vi "replace plot - plot ref - V2.vi"(0 "Plot ref in":refnum<vi>, 1 "Array X IN":dbl[](array[numeric]), 2 "Array Y IN":dbl[](array[numeric]), 5 "plot index":i32, 6 "cursor action":T2=enum."write", 7 "label":enum16{"hide", "show x", "show y", "show (x,y)"}(ring), 12 "Color Box":u32(colorbox)=327424, 13 "cursor state":T3=enum."boring") -> (14 "Plot ref out":refnum<vi>, 15 "Array X":dbl[](array[numeric]), 16 "Array Y":dbl[](array[numeric]), 19 "2Dwindow bounds out":T1={"min y"=0.0021014740628288917, "max x"=44850.89441339177, "min x"=2.5658109925320947, "max y"=17480.201988350764} {"max y" format="%#9_9f"; "min x" format="%#9_9f"; "max x" format="%#9_9f"})   [LabVIEW 2020]
uses:
  cursor sate.ctl
  cursor action.ctl
  2Dwindow-bounds.ctl
  stack action -- control.ctl
  range multiplier action.ctl
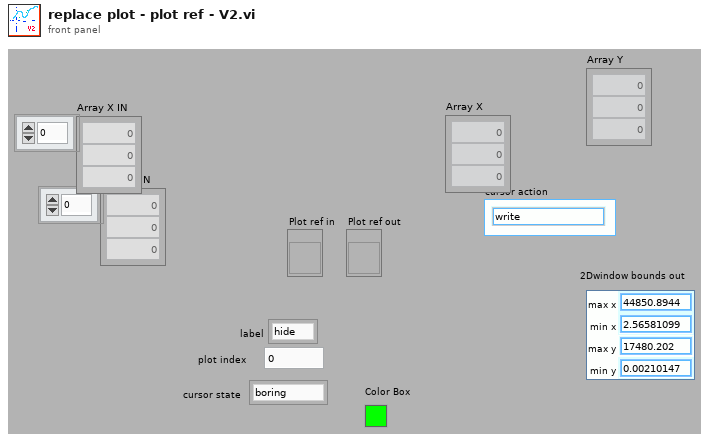
[diagram p1: front panel]
types:
  T1 = typedef "2Dwindow-bounds.ctl" = cluster{"min y":dbl, "max x":dbl, "min x":dbl, "max y":dbl}
  T2 = typedef "cursor action.ctl" = enum16{"range", "read", "write", "check", "zoom out", "smart zoom out", "zoom to aspect ratio 1", "zoom to win", "zoom out 20%", "zoom in 20%", "-empty", "smart zoom out&aspect", "move range left 20%", "move range right 20%", "move range up 20%", "move range down 20%", "zoom to X win", "zoom to Y win", "zoom out X", "zoom out Y", "zoom in X", "zoom in Y", "check plot scale", "set color"}
  T3 = typedef "cursor sate.ctl" = enum16{"normal", "alert", "fuzzy", "interesting", "boring", "colored"}
  T4 = typedef "stack action -- control.ctl" = enum16{"push", "pop", "check", "init"}
  T5 = typedef "range multiplier action.ctl" = enum16{"shift", "zoom", "check"}
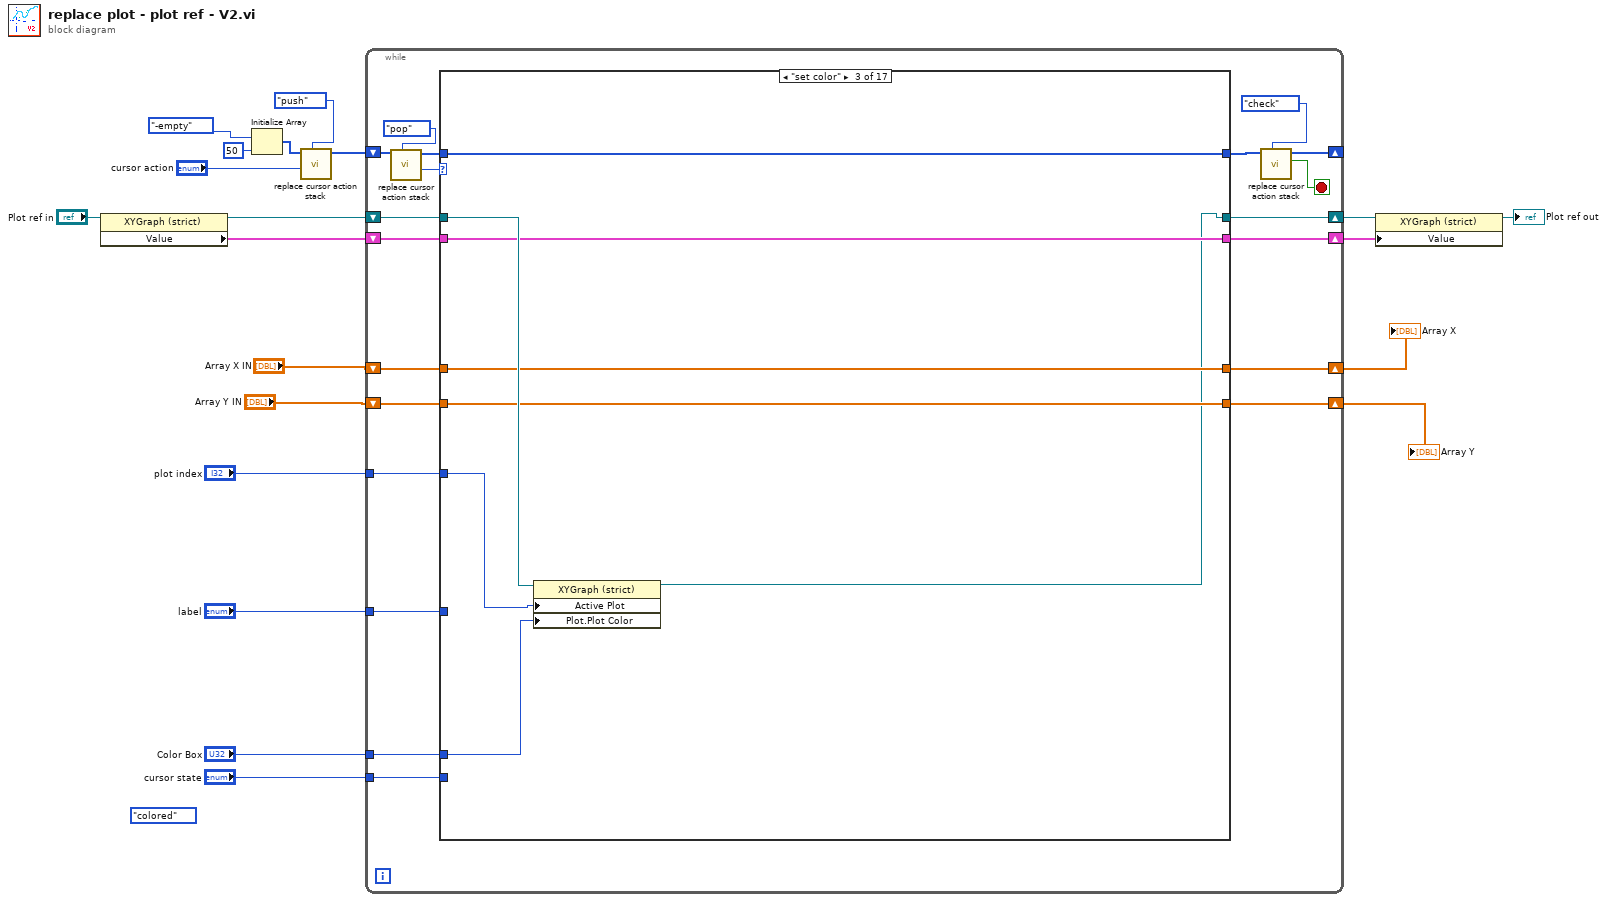
[diagram p0: block diagram]
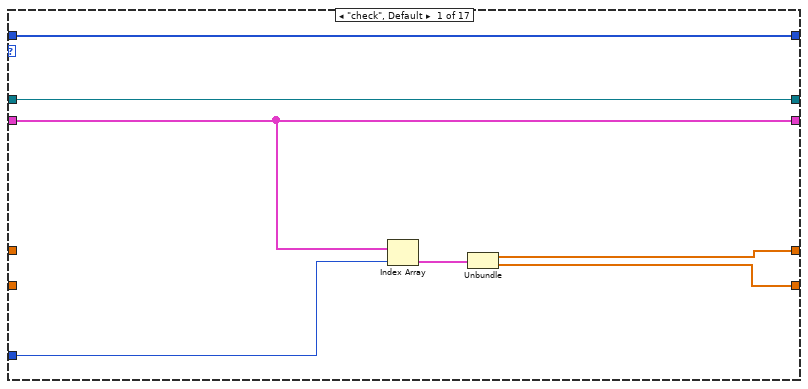
[diagram p2: hidden frame]
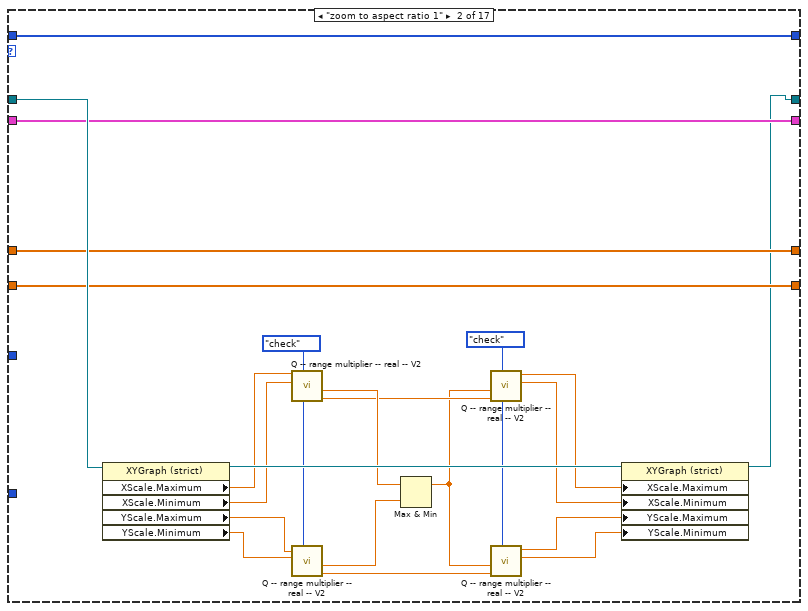
[diagram p3: hidden frame]
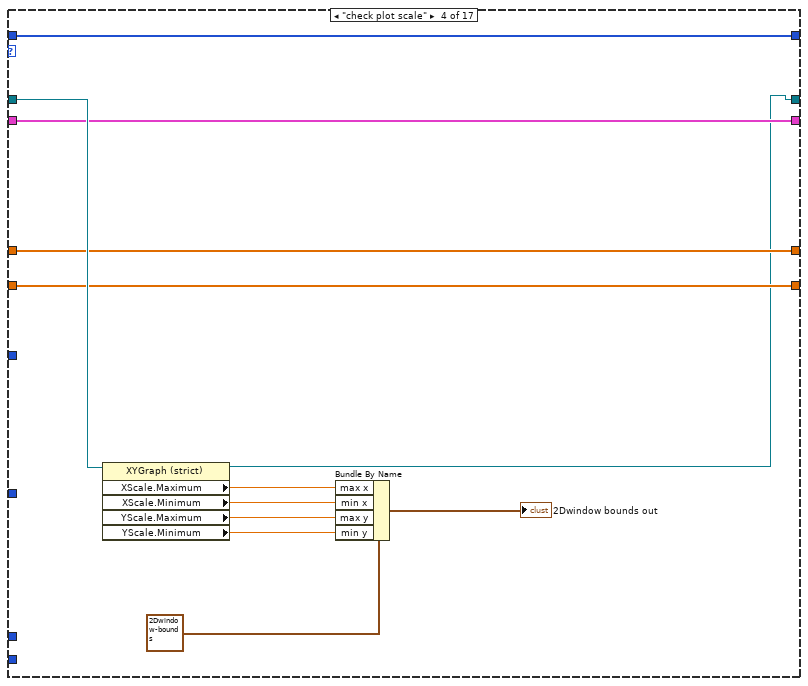
[diagram p4: hidden frame]
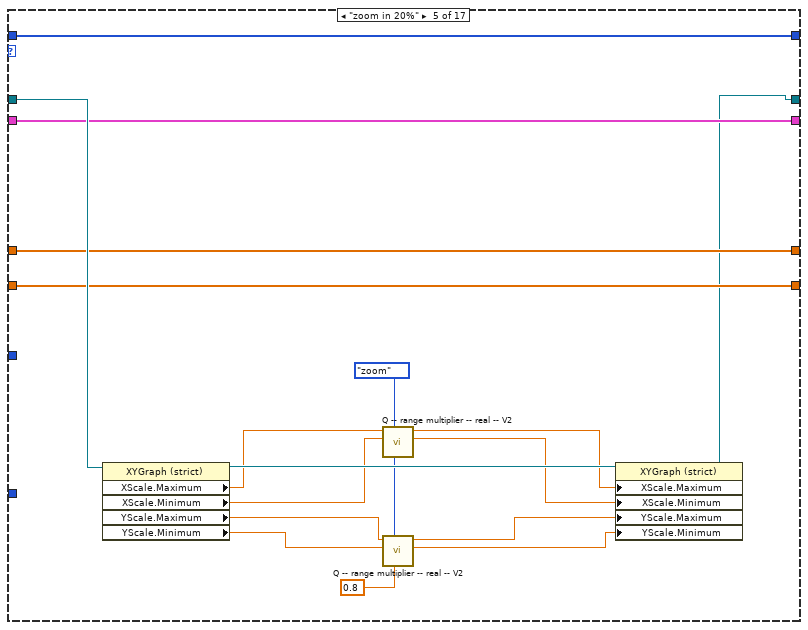
[diagram p5: hidden frame]
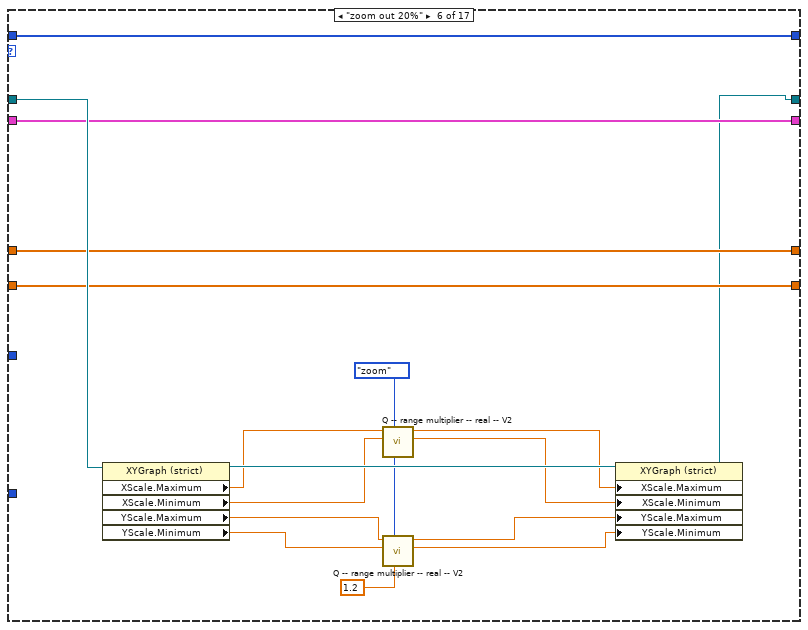
[diagram p6: hidden frame]
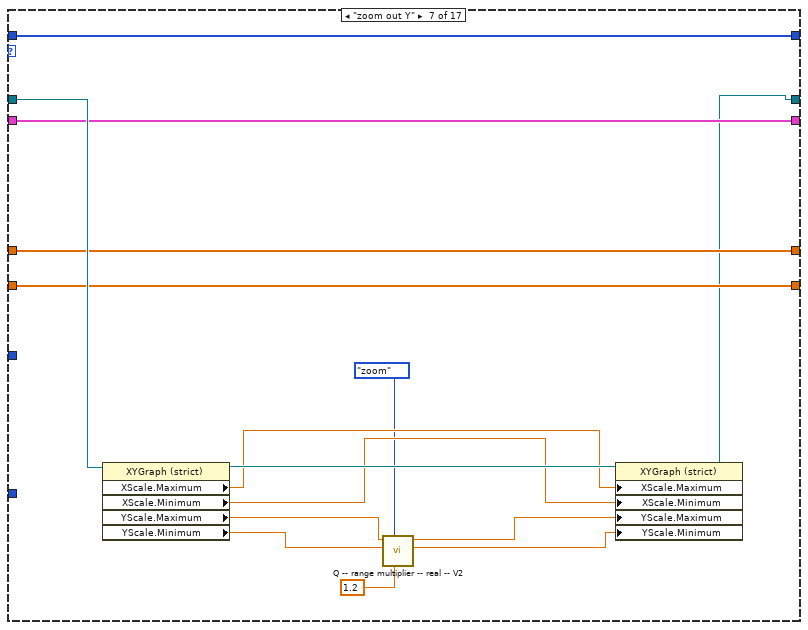
[diagram p7: hidden frame]
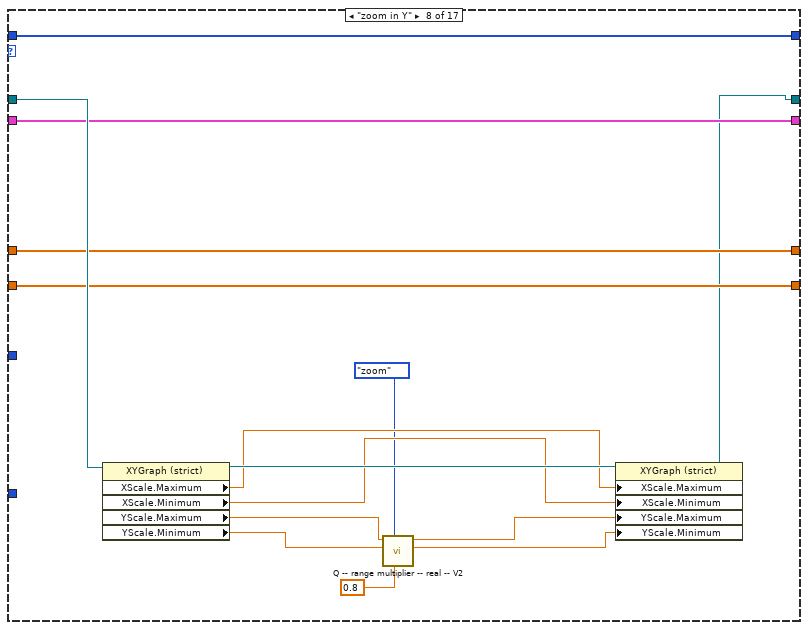
[diagram p8: hidden frame]
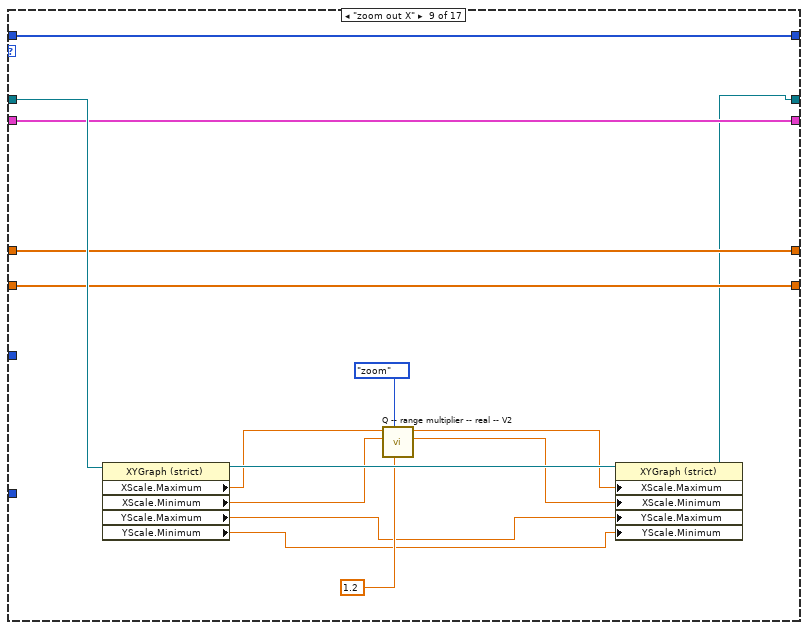
[diagram p9: hidden frame]
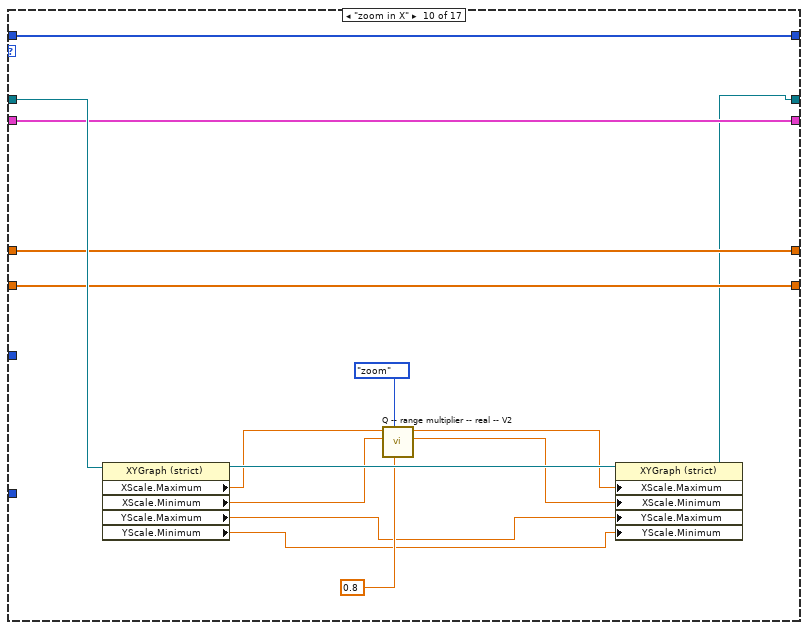
[diagram p10: hidden frame]
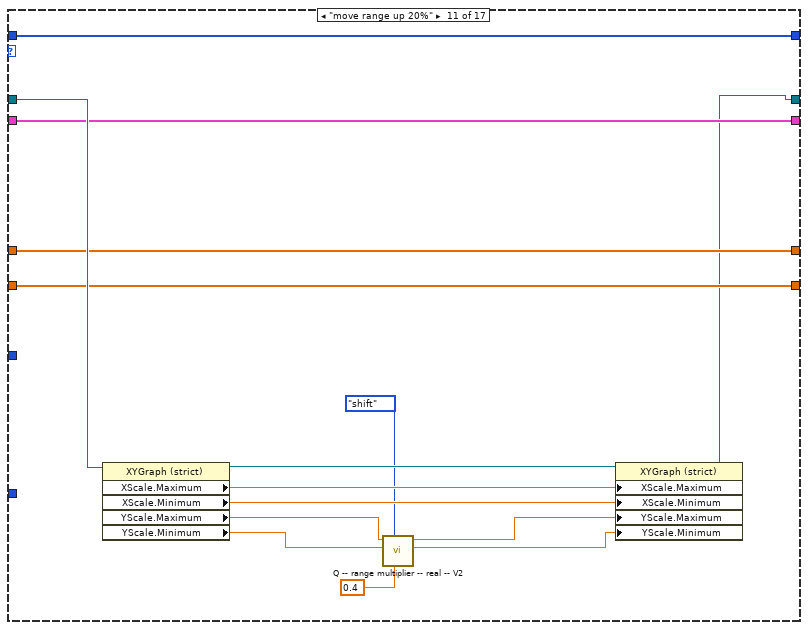
[diagram p11: hidden frame]
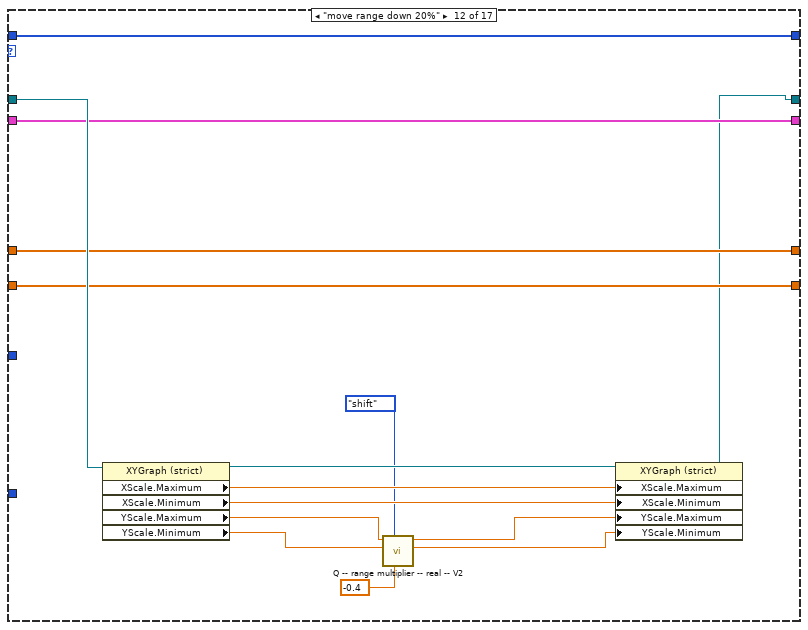
[diagram p12: hidden frame]
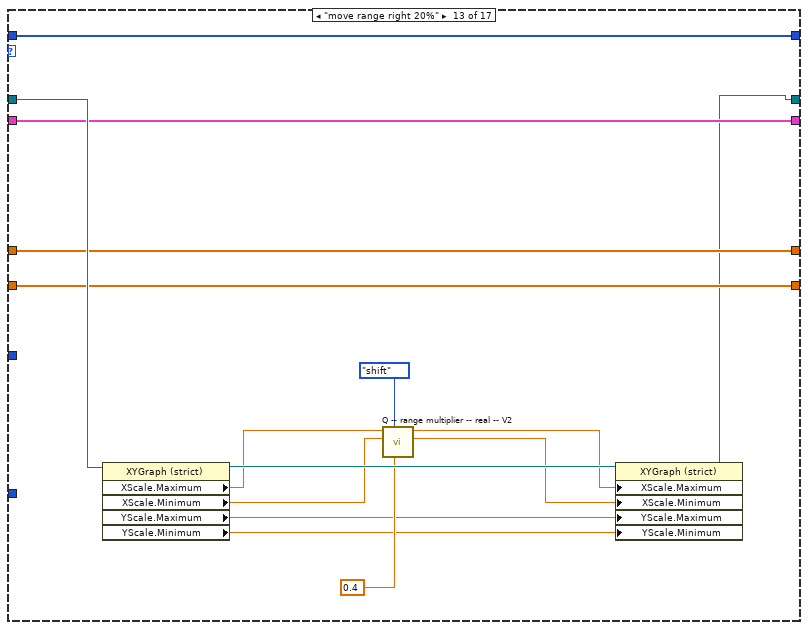
[diagram p13: hidden frame]
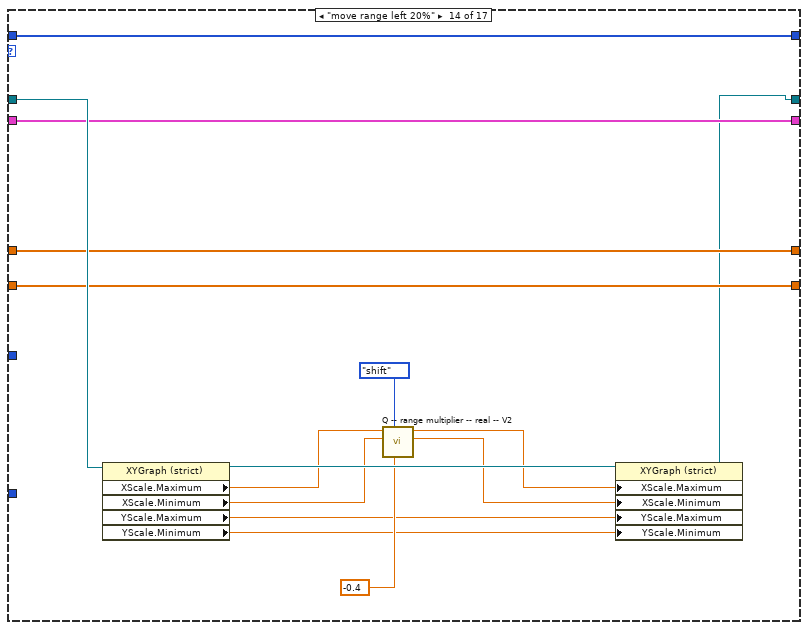
[diagram p14: hidden frame]
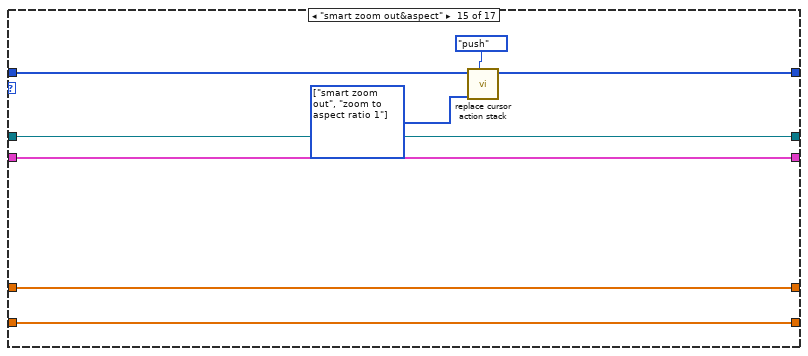
[diagram p15: hidden frame]
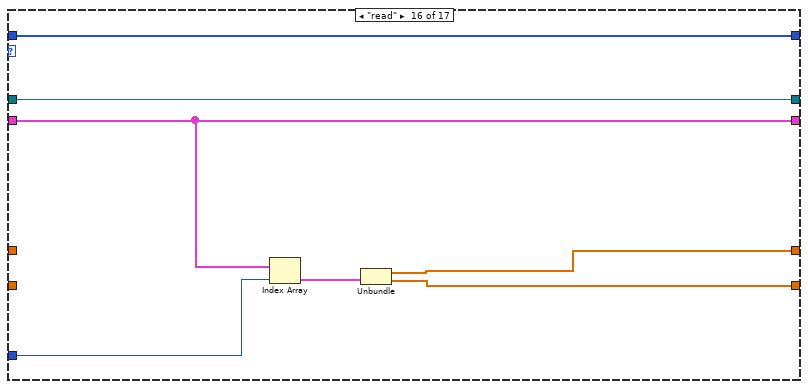
[diagram p16: hidden frame]
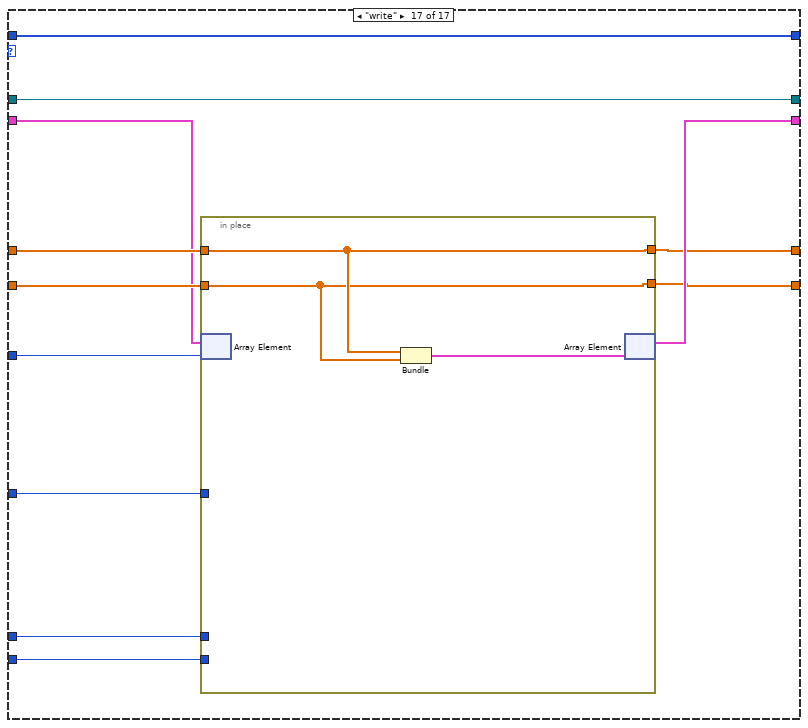
[diagram p17: hidden frame]
diagram:
  (unwired) cursor_sate."colored" ("cursor state")
  n1 = property on="Property Node" class="XYGraph (strict)"(reference="Plot ref in") -> (reference out=w12:refnum<vi>, "Value"=w19:cluster{dbl[], dbl[]}[])  [unwired: 1 in, 1 out]
  n2 = Initialize Array(cursor_action."-empty" ("cursor action"), 50 ("dimension size")) -> (w8:T2[])
  n3 = call "replace cursor action stack.vi"("stack action"=stack_action_--_control."push", "cursor action"="cursor action", "command stack In"=w8) -> ("command stack Out"=w5:T2[])  [unwired: 6 in, 2 out]
  n4 = while {
    tunnel: "plot index" -> [w40]
    tunnel: "label" -> [w36]
    tunnel: "Color Box" -> [w35]
    tunnel: "cursor state" -> [w34]
    shift-right: [w31] -> w11
    shift-left: w19 -> [w37]
    shift-right: [w33] -> w13
    shift-left: w12 -> [w32]
    shift-right: [w26] -> _
    shift-left: w5 -> [w30]
    shift-right: [w23] -> w3
    shift-left: "Array Y IN" -> [w39]
    shift-right: [w22] -> w4
    shift-left: "Array X IN" -> [w38]
    stop <- w27 stop-if-true
    n5 = call "replace cursor action stack.vi"("stack action"=stack_action_--_control."pop", "command stack In"=w30) -> ("cursor action Out"=w28:T2, "command stack Out"=w24:T2[])  [unwired: 7 in, 1 out]
    n6 = case shown="\"set color\"" w28 {
      tunnel: w40 -> [w45 _ w72 _ _ _ _ _ _ _ _ _ _ _ _ w258 w266]
      tunnel: w37 -> [w46 w67 w76 w88 w104 w121 w136 w151 w166 w181 w196 w211 w226 w241 w244 w257 w268]
      tunnel: w39 -> [_ w65 w74 w86 w102 w119 w134 w149 w164 w179 w194 w209 w224 w239 w246 _ w269]
      tunnel: w38 -> [_ w66 w75 w87 w103 w120 w135 w150 w165 w180 w195 w210 w225 w240 w247 _ w270]
      tunnel: [w42 w66 w75 w87 w103 w120 w135 w150 w165 w180 w195 w210 w225 w240 w247 w253 w265] -> w22
      tunnel: [w41 w65 w74 w86 w102 w119 w134 w149 w164 w179 w194 w209 w224 w239 w246 w252 w264] -> w23
      tunnel: w36 -> [_ _ _ _ _ _ _ _ _ _ _ _ _ _ _ _ w263]
      tunnel: w35 -> [_ _ w71 _ _ _ _ _ _ _ _ _ _ _ _ _ w262]
      tunnel: w34 -> [_ _ _ _ _ _ _ _ _ _ _ _ _ _ _ _ w261]
      tunnel: [w47 w63 w70 w84 w100 w117 w132 w147 w162 w177 w192 w207 w222 w237 w245 w256 w260] -> w33
      tunnel: w32 -> [w47 w68 w77 w89 w105 w122 w137 w152 w167 w182 w197 w212 w227 w242 w245 w256 w260]
      tunnel: [w46 w67 w76 w88 w104 w121 w136 w151 w166 w181 w196 w211 w226 w241 w244 w257 w267] -> w31
      tunnel: [w44 w64 w73 w85 w101 w118 w133 w148 w163 w178 w193 w208 w223 w238 w249 w255 w259] -> w25
      tunnel: w24 -> [w44 w64 w73 w85 w101 w118 w133 w148 w163 w178 w193 w208 w223 w238 w250 w255 w259]
      frame "check", Default {
        n7 = Index Array(array=w46, index=w45) -> (element=w43:cluster{dbl[], dbl[]})
        n8 = Unbundle(w43) -> (w42:dbl[], w41:dbl[])
      }
      frame "zoom to aspect ratio 1" {
        w52 = range_multiplier_action."check" ("rage multiplier action")
        w58 = range_multiplier_action."check" ("rage multiplier action")
        n9 = property on="Property Node" class="XYGraph (strict)"(reference=w68) -> (reference out=w69:refnum<vi>, "XScale.Maximum"=w62:dbl, "XScale.Minimum"=w61:dbl, "YScale.Maximum"=w60:dbl, "YScale.Minimum"=w59:dbl)  [unwired: 1 in, 1 out]
        n10 = call "Q -- range multiplier -- real -- V2.vi"("rage multiplier action"=w58, "lower"=w61, "upper"=w62) -> ("center OUT"=w55:dbl, "window OUT"=w57:dbl)  [unwired: 5 in, 2 out]
        n11 = call "Q -- range multiplier -- real -- V2.vi"("rage multiplier action"=w58, "lower"=w59, "upper"=w60) -> ("center OUT"=w54:dbl, "window OUT"=w56:dbl)  [unwired: 5 in, 2 out]
        n12 = Max & Min(x=w57, y=w56) -> (max(x,y)=w53:dbl)  [unwired: 1 out]
        n13 = call "Q -- range multiplier -- real -- V2.vi"("rage multiplier action"=w52, "center"=w55, "window"=w53) -> ("lower OUT"=w48:dbl, "upper OUT"=w49:dbl)  [unwired: 5 in, 2 out]
        n14 = call "Q -- range multiplier -- real -- V2.vi"("rage multiplier action"=w52, "center"=w54, "window"=w53) -> ("lower OUT"=w50:dbl, "upper OUT"=w51:dbl)  [unwired: 5 in, 2 out]
        n15 = property on="Property Node" class="XYGraph (strict)"(reference=w69, "XScale.Maximum"=w49, "XScale.Minimum"=w48, "YScale.Maximum"=w51, "YScale.Minimum"=w50) -> (reference out=w63:refnum<vi>)  [unwired: 1 in, 1 out]
      }
      frame "set color" {
        n16 = property on="Property Node" class="XYGraph (strict)"(reference=w77, "Active Plot"=w72, "Plot.Plot Color"=w71) -> (reference out=w70:refnum<vi>)  [unwired: 1 in, 1 out]
      }
      frame "check plot scale" {
        n17 = property on="Property Node" class="XYGraph (strict)"(reference=w89) -> (reference out=w84:refnum<vi>, "XScale.Maximum"=w82:dbl, "XScale.Minimum"=w81:dbl, "YScale.Maximum"=w80:dbl, "YScale.Minimum"=w79:dbl)  [unwired: 1 in, 1 out]
        n18 = Bundle By Name(cluster=T1 {"min y"=0.0021014740628288917, "max x"=44850.89441339177, "min x"=2.5658109925320947, "max y"=17480.201988350764} ("2Dwindow bounds out"), "max x"=w82, "min x"=w81, "max y"=w80, "min y"=w79) -> (→"2Dwindow bounds out":T1)
      }
      frame "zoom in 20%" {
        w91 = range_multiplier_action."zoom" ("rage multiplier action")
        w90 = 0.8
        n19 = property on="Property Node" class="XYGraph (strict)"(reference=w105) -> (reference out=w106:refnum<vi>, "XScale.Maximum"=w99:dbl, "XScale.Minimum"=w98:dbl, "YScale.Maximum"=w95:dbl, "YScale.Minimum"=w94:dbl)  [unwired: 1 in, 1 out]
        n20 = call "Q -- range multiplier -- real -- V2.vi"("factor"=w90, "rage multiplier action"=w91, "lower"=w98, "upper"=w99) -> ("lower OUT"=w96:dbl, "upper OUT"=w97:dbl)  [unwired: 4 in, 2 out]
        n21 = call "Q -- range multiplier -- real -- V2.vi"("factor"=w90, "rage multiplier action"=w91, "lower"=w94, "upper"=w95) -> ("lower OUT"=w92:dbl, "upper OUT"=w93:dbl)  [unwired: 4 in, 2 out]
        n22 = property on="Property Node" class="XYGraph (strict)"(reference=w106, "XScale.Maximum"=w97, "XScale.Minimum"=w96, "YScale.Maximum"=w93, "YScale.Minimum"=w92) -> (reference out=w100:refnum<vi>)  [unwired: 1 in, 1 out]
      }
      frame "zoom out 20%" {
        w108 = range_multiplier_action."zoom" ("rage multiplier action")
        w107 = 1.2
        n23 = property on="Property Node" class="XYGraph (strict)"(reference=w122) -> (reference out=w123:refnum<vi>, "XScale.Maximum"=w116:dbl, "XScale.Minimum"=w115:dbl, "YScale.Maximum"=w112:dbl, "YScale.Minimum"=w111:dbl)  [unwired: 1 in, 1 out]
        n24 = call "Q -- range multiplier -- real -- V2.vi"("factor"=w107, "rage multiplier action"=w108, "lower"=w115, "upper"=w116) -> ("lower OUT"=w113:dbl, "upper OUT"=w114:dbl)  [unwired: 4 in, 2 out]
        n25 = call "Q -- range multiplier -- real -- V2.vi"("factor"=w107, "rage multiplier action"=w108, "lower"=w111, "upper"=w112) -> ("lower OUT"=w109:dbl, "upper OUT"=w110:dbl)  [unwired: 4 in, 2 out]
        n26 = property on="Property Node" class="XYGraph (strict)"(reference=w123, "XScale.Maximum"=w114, "XScale.Minimum"=w113, "YScale.Maximum"=w110, "YScale.Minimum"=w109) -> (reference out=w117:refnum<vi>)  [unwired: 1 in, 1 out]
      }
      frame "zoom out Y" {
        n27 = property on="Property Node" class="XYGraph (strict)"(reference=w137) -> (reference out=w138:refnum<vi>, "XScale.Maximum"=w126:dbl, "XScale.Minimum"=w125:dbl, "YScale.Maximum"=w131:dbl, "YScale.Minimum"=w130:dbl)  [unwired: 1 in, 1 out]
        n28 = call "Q -- range multiplier -- real -- V2.vi"("factor"=1.2, "rage multiplier action"=range_multiplier_action."zoom", "lower"=w130, "upper"=w131) -> ("lower OUT"=w128:dbl, "upper OUT"=w129:dbl)  [unwired: 4 in, 2 out]
        n29 = property on="Property Node" class="XYGraph (strict)"(reference=w138, "XScale.Maximum"=w126, "XScale.Minimum"=w125, "YScale.Maximum"=w129, "YScale.Minimum"=w128) -> (reference out=w132:refnum<vi>)  [unwired: 1 in, 1 out]
      }
      frame "zoom in Y" {
        n30 = property on="Property Node" class="XYGraph (strict)"(reference=w152) -> (reference out=w153:refnum<vi>, "XScale.Maximum"=w141:dbl, "XScale.Minimum"=w140:dbl, "YScale.Maximum"=w146:dbl, "YScale.Minimum"=w145:dbl)  [unwired: 1 in, 1 out]
        n31 = call "Q -- range multiplier -- real -- V2.vi"("factor"=0.8, "rage multiplier action"=range_multiplier_action."zoom", "lower"=w145, "upper"=w146) -> ("lower OUT"=w143:dbl, "upper OUT"=w144:dbl)  [unwired: 4 in, 2 out]
        n32 = property on="Property Node" class="XYGraph (strict)"(reference=w153, "XScale.Maximum"=w141, "XScale.Minimum"=w140, "YScale.Maximum"=w144, "YScale.Minimum"=w143) -> (reference out=w147:refnum<vi>)  [unwired: 1 in, 1 out]
      }
      frame "zoom out X" {
        n33 = property on="Property Node" class="XYGraph (strict)"(reference=w167) -> (reference out=w168:refnum<vi>, "XScale.Maximum"=w161:dbl, "XScale.Minimum"=w160:dbl, "YScale.Maximum"=w155:dbl, "YScale.Minimum"=w154:dbl)  [unwired: 1 in, 1 out]
        n34 = call "Q -- range multiplier -- real -- V2.vi"("factor"=1.2, "rage multiplier action"=range_multiplier_action."zoom", "lower"=w160, "upper"=w161) -> ("lower OUT"=w158:dbl, "upper OUT"=w159:dbl)  [unwired: 4 in, 2 out]
        n35 = property on="Property Node" class="XYGraph (strict)"(reference=w168, "XScale.Maximum"=w159, "XScale.Minimum"=w158, "YScale.Maximum"=w155, "YScale.Minimum"=w154) -> (reference out=w162:refnum<vi>)  [unwired: 1 in, 1 out]
      }
      frame "zoom in X" {
        n36 = property on="Property Node" class="XYGraph (strict)"(reference=w182) -> (reference out=w183:refnum<vi>, "XScale.Maximum"=w176:dbl, "XScale.Minimum"=w175:dbl, "YScale.Maximum"=w170:dbl, "YScale.Minimum"=w169:dbl)  [unwired: 1 in, 1 out]
        n37 = call "Q -- range multiplier -- real -- V2.vi"("factor"=0.8, "rage multiplier action"=range_multiplier_action."zoom", "lower"=w175, "upper"=w176) -> ("lower OUT"=w173:dbl, "upper OUT"=w174:dbl)  [unwired: 4 in, 2 out]
        n38 = property on="Property Node" class="XYGraph (strict)"(reference=w183, "XScale.Maximum"=w174, "XScale.Minimum"=w173, "YScale.Maximum"=w170, "YScale.Minimum"=w169) -> (reference out=w177:refnum<vi>)  [unwired: 1 in, 1 out]
      }
      frame "move range up 20%" {
        n39 = property on="Property Node" class="XYGraph (strict)"(reference=w197) -> (reference out=w198:refnum<vi>, "XScale.Maximum"=w185:dbl, "XScale.Minimum"=w186:dbl, "YScale.Maximum"=w191:dbl, "YScale.Minimum"=w190:dbl)  [unwired: 1 in, 1 out]
        n40 = call "Q -- range multiplier -- real -- V2.vi"("factor"=0.4, "rage multiplier action"=range_multiplier_action."shift", "lower"=w190, "upper"=w191) -> ("lower OUT"=w188:dbl, "upper OUT"=w189:dbl)  [unwired: 4 in, 2 out]
        n41 = property on="Property Node" class="XYGraph (strict)"(reference=w198, "XScale.Maximum"=w185, "XScale.Minimum"=w186, "YScale.Maximum"=w189, "YScale.Minimum"=w188) -> (reference out=w192:refnum<vi>)  [unwired: 1 in, 1 out]
      }
      frame "move range down 20%" {
        n42 = property on="Property Node" class="XYGraph (strict)"(reference=w212) -> (reference out=w213:refnum<vi>, "XScale.Maximum"=w200:dbl, "XScale.Minimum"=w201:dbl, "YScale.Maximum"=w206:dbl, "YScale.Minimum"=w205:dbl)  [unwired: 1 in, 1 out]
        n43 = call "Q -- range multiplier -- real -- V2.vi"("factor"=-0.4, "rage multiplier action"=range_multiplier_action."shift", "lower"=w205, "upper"=w206) -> ("lower OUT"=w203:dbl, "upper OUT"=w204:dbl)  [unwired: 4 in, 2 out]
        n44 = property on="Property Node" class="XYGraph (strict)"(reference=w213, "XScale.Maximum"=w200, "XScale.Minimum"=w201, "YScale.Maximum"=w204, "YScale.Minimum"=w203) -> (reference out=w207:refnum<vi>)  [unwired: 1 in, 1 out]
      }
      frame "move range right 20%" {
        n45 = property on="Property Node" class="XYGraph (strict)"(reference=w227) -> (reference out=w228:refnum<vi>, "XScale.Maximum"=w221:dbl, "XScale.Minimum"=w220:dbl, "YScale.Maximum"=w215:dbl, "YScale.Minimum"=w214:dbl)  [unwired: 1 in, 1 out]
        n46 = call "Q -- range multiplier -- real -- V2.vi"("factor"=0.4, "rage multiplier action"=range_multiplier_action."shift", "lower"=w220, "upper"=w221) -> ("lower OUT"=w218:dbl, "upper OUT"=w219:dbl)  [unwired: 4 in, 2 out]
        n47 = property on="Property Node" class="XYGraph (strict)"(reference=w228, "XScale.Maximum"=w219, "XScale.Minimum"=w218, "YScale.Maximum"=w215, "YScale.Minimum"=w214) -> (reference out=w222:refnum<vi>)  [unwired: 1 in, 1 out]
      }
      frame "move range left 20%" {
        n48 = property on="Property Node" class="XYGraph (strict)"(reference=w242) -> (reference out=w243:refnum<vi>, "XScale.Maximum"=w236:dbl, "XScale.Minimum"=w235:dbl, "YScale.Maximum"=w230:dbl, "YScale.Minimum"=w229:dbl)  [unwired: 1 in, 1 out]
        n49 = call "Q -- range multiplier -- real -- V2.vi"("factor"=-0.4, "rage multiplier action"=range_multiplier_action."shift", "lower"=w235, "upper"=w236) -> ("lower OUT"=w233:dbl, "upper OUT"=w234:dbl)  [unwired: 4 in, 2 out]
        n50 = property on="Property Node" class="XYGraph (strict)"(reference=w243, "XScale.Maximum"=w234, "XScale.Minimum"=w233, "YScale.Maximum"=w230, "YScale.Minimum"=w229) -> (reference out=w237:refnum<vi>)  [unwired: 1 in, 1 out]
      }
      frame "smart zoom out&aspect" {
        w248 = T2[] [enum."smart zoom out", enum."zoom to aspect ratio 1"] items=["range", "read", "write", "check", "zoom out", "smart zoom out", "zoom to aspect ratio 1", "zoom to win", "zoom out 20%", "zoom in 20%", "-empty", "smart zoom out&aspect", "move range left 20%", "move range right 20%", "move range up 20%", "move range down 20%", "zoom to X win", "zoom to Y win", "zoom out X", "zoom out Y", "zoom in X", "zoom in Y", "check plot scale", "set color"] ("action list I")
        n51 = call "replace cursor action stack.vi"("stack action"=stack_action_--_control."push", "action list I"=w248, "command stack In"=w250) -> ("command stack Out"=w249:T2[])  [unwired: 6 in, 2 out]
      }
      frame "read" {
        n52 = Index Array(array=w257, index=w258) -> (element=w254:cluster{dbl[], dbl[]})
        n53 = Unbundle(w254) -> (w253:dbl[], w252:dbl[])
      }
      frame "write" {
        n54 = in-place {
          in-place-border: w270 -> [w273]
          in-place-border: w269 -> [w272]
          in-place-border: [w273] -> w265
          in-place-border: [w272] -> w264
          in-place-border: w263 -> [_]
          in-place-border: w262 -> [_]
          in-place-border: w261 -> [_]
          n55 = in-place-array #1(w268, w266) -> ()  [unwired: 1 out]
          n56 = Bundle("Array X IN"=w273, "Array Y IN"=w272) -> (w271:cluster{"Array X IN":dbl[], "Array Y IN":dbl[]})  [unwired: 1 in]
          n57 = in-place-array #1(w271) -> (w267:cluster{dbl[], dbl[]}[])  [unwired: 1 out]
        }
      }
    }
    n58 = call "replace cursor action stack.vi"("stack action"=stack_action_--_control."check", "command stack In"=w25) -> ("stack is empty ?"=w27:bool, "command stack Out"=w26:T2[])  [unwired: 7 in, 1 out]
  }
  "Array X" <- w4
  "Array Y" <- w3
  n59 = property on="Property Node" class="XYGraph (strict)"(reference=w13, "Value"=w11) -> (reference out=→"Plot ref out":refnum<vi>)  [unwired: 1 in, 1 out]
